vi "readFromXML.vi"(8 "error in (no error)":errorcluster, 10 "XML in":string, 11 "MccRotStop in":refnum<class "MccRotStop.lvclass">) -> (0 "error out":errorcluster, 3 "MccRotStop out":refnum<class "MccRotStop.lvclass">)   [LabVIEW 2014, in "TCSDataDefinitions.lvlib" / "TCSMountControlCommand.lvlib" / "CommandsForRotatorAxis.lvlib" / "MccRotStop.lvclass"]
uses:
  MccRotStop.lvclass
  CommandsForRotatorAxis.lvclass
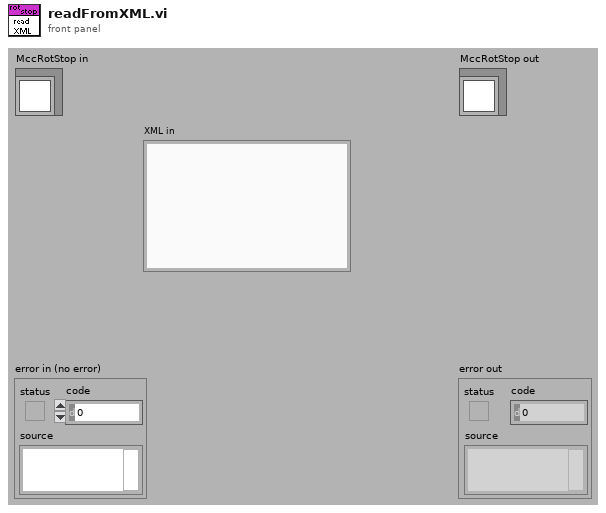
[diagram p1: front panel]
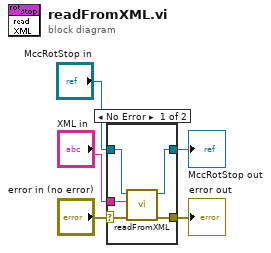
[diagram p0: block diagram]
diagram:
  n1 = case shown="No Error" "error in (no error)" {
    selector: "error in (no error)" -> [w7 w12]
    tunnel: [w6 w12] -> w4
    tunnel: [w8 w11] -> w2
    tunnel: "MccRotStop in" -> [w9 w11]
    tunnel: "XML in" -> [w10 _]
    frame No Error {
      n2 = call-parent "readFromXML.vi"("error in (no error)"=w7, "XML in"=w10, "CommandsForRotatorAxis in"=w9) -> ("error out"=w6:errorcluster, "CommandsForRotatorAxis out"=w8:refnum<class "MccRotStop.lvclass">)  [unwired: 7 out]
    }
    frame Error {
    }
  }
  "error out" <- w4
  "MccRotStop out" <- w2
